vi "限幅器（U8）.vi"(3 "下限":u8, 4 "X_in":u8, 5 "上限":u8) -> (1 "X_Out":u8)   [LabVIEW 2012]
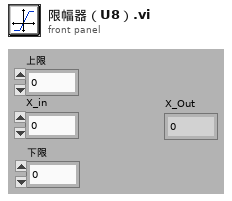
[diagram p1: front panel]
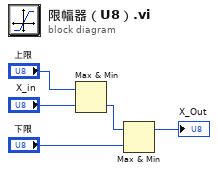
[diagram p0: block diagram]
diagram:
  n1 = Max & Min(x="上限", y="X_in") -> (min(x,y)=w3:u8)  [unwired: 1 out]
  n2 = Max & Min(x=w3, y="下限") -> (max(x,y)=→"X_Out":u8)  [unwired: 1 out]
